vi "Next value.vi"(8 "error in (no error)":errorcluster, 9 "timeout":dbl[unit]=1.0, 11 "Subscription in":refnum<class "Subscription.lvclass">) -> (0 "error out":errorcluster, 1 "timed out?":bool, 2 "value":refnum<class "Value.lvclass">, 3 "Subscription out":refnum<class "Subscription.lvclass">, 5 "PV name":string)   [LabVIEW 2020, in "Client.lvlib" / "Subscription.lvclass"]
uses:
  Subscription.lvclass
  Value/Value/Value.lvclass
  Subscription.lvclass/Subscription.ctl
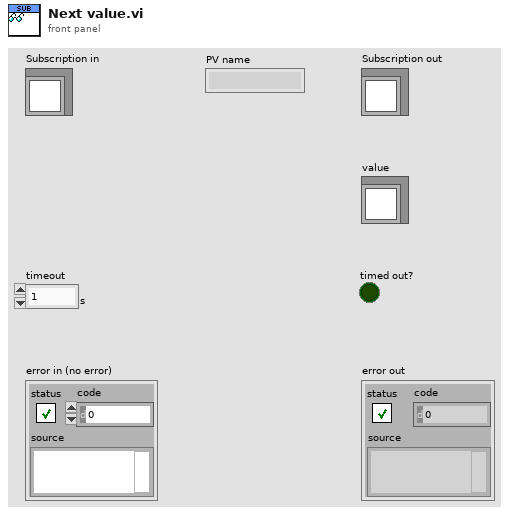
[diagram p1: front panel]
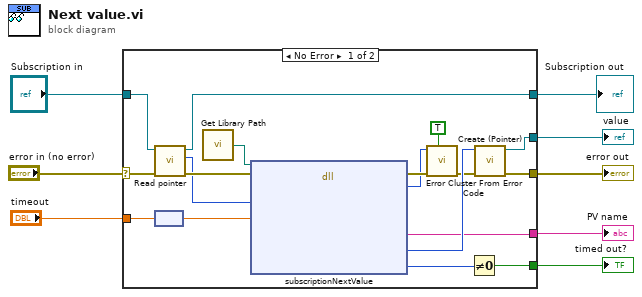
[diagram p0: block diagram]
diagram:
  n1 = case shown="No Error" "error in (no error)" {
    selector: "error in (no error)" -> [w23 w27]
    tunnel: [w26 w27] -> w7
    tunnel: [w20 w28] -> w5
    tunnel: "Subscription in" -> [w21 w28]
    tunnel: "timeout" -> [w14 _]
    tunnel: [w25 _] -> w4
    tunnel: [w16 _] -> w3
    tunnel: [w9 _] -> w1
    frame No Error {
      n2 = call "Read pointer.vi"("error in (no error)"=w23, "Subscription in"=w21) -> ("error out"=w22:errorcluster, "pointer"=w19:i64, "Subscription out"=w20:refnum<class "Subscription.lvclass">)  [unwired: 7 in]
      n3 = node(w14) -> (w15:dbl)
      n4 = call "Get Library Path.vi"() -> ("Path"=w24:path)  [unwired: 1 in]
      n5 = dll-call lib="?" fn="subscriptionNextValue"(path in=w24, error in=w22, "subscription"=w19, "timeout"=w15) -> (error out=w12:errorcluster, "ret_code"=w10:i32, "pvName"=w9:string, "value"=w18:i64, "timedOut"=w17:i16)  [unwired: 6 in, 1 out]
      n6 = call <vilib>:"Error Cluster From Error Code.vi"("show call chain? (False)"=TRUE, "error in (no error)"=w12, "error code (0)"=w10) -> ("error out"=w11:errorcluster)  [unwired: 6 in]
      n7 = Not Equal To 0?(x=w17) -> (x != 0?=w16:bool)
      n8 = call "Create (Pointer).vi"("error in"=w11, "pointer"=w18) -> ("error out"=w26:errorcluster, "Value out"=w25:refnum<class "Value.lvclass">)  [unwired: 8 in]
    }
    frame Error {
    }
  }
  "error out" <- w7
  "Subscription out" <- w5
  "timed out?" <- w3
  "value" <- w4
  "PV name" <- w1
